vi "Zernike_Mode_Boolean_Selector_v01.vi"(0 "1st  Spherical Aberration":bool, 1 "2nd Spherical Aberration":bool, 2 "Oblique Astigmatism":bool, 3 "Vertical Astigmatism":bool, 4 "Horizontal Coma":bool, 5 "Vertical Coma":bool) -> (14 "ZM 1":i32[](array[numeric]), 15 "ZM 2":i32[](array[numeric]))   [LabVIEW 2015]
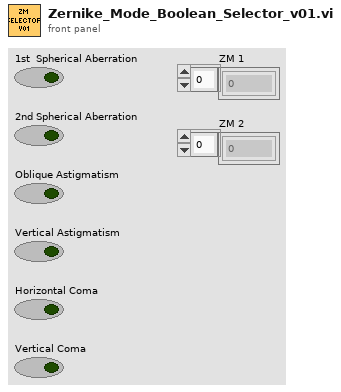
[diagram p1: front panel]
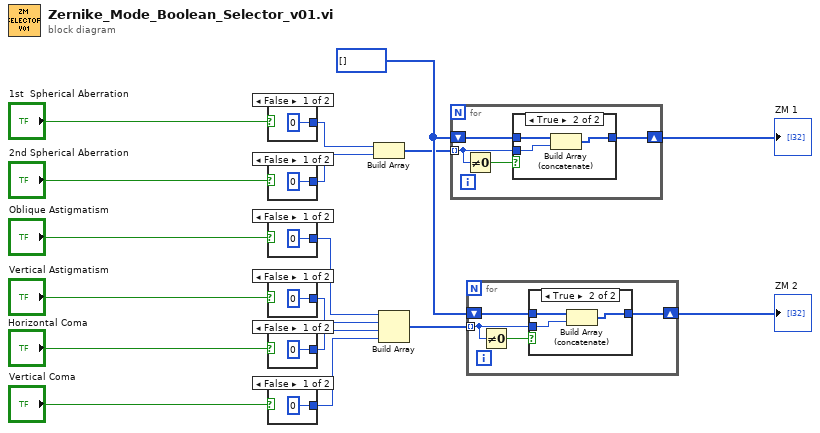
[diagram p0: block diagram]
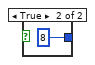
[diagram p4: hidden frame]
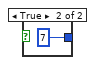
[diagram p5: hidden frame]
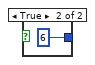
[diagram p6: hidden frame]
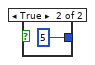
[diagram p7: hidden frame]
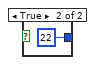
[diagram p8: hidden frame]
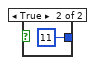
[diagram p9: hidden frame]
diagram:
  w16 = i32[] []
  n1 = case shown="False" "1st  Spherical Aberration" {
    tunnel: [0 11] -> w7
    frame False {
    }
    frame True {
    }
  }
  n2 = case shown="False" "2nd Spherical Aberration" {
    tunnel: [0 22] -> w8
    frame False {
    }
    frame True {
    }
  }
  n3 = case shown="False" "Oblique Astigmatism" {
    tunnel: [0 5] -> w9
    frame False {
    }
    frame True {
    }
  }
  n4 = case shown="False" "Vertical Astigmatism" {
    tunnel: [0 6] -> w10
    frame False {
    }
    frame True {
    }
  }
  n5 = case shown="False" "Horizontal Coma" {
    tunnel: [0 7] -> w11
    frame False {
    }
    frame True {
    }
  }
  n6 = case shown="False" "Vertical Coma" {
    tunnel: [0 8] -> w12
    frame False {
    }
    frame True {
    }
  }
  n7 = Build Array(w7, w8) -> (w13:i32[])
  n8 = Build Array(w9, w10, w11, w12) -> (w17:i32[])
  n9 = for {
    tunnel: w13 -> [w32] mode=indexing
    shift-right: [w30] -> w14
    shift-left: w16 -> [w31]
    n10 = Not Equal To 0?(x=w32) -> (x != 0?=w33:bool)
    n11 = case shown="True" w33 {
      tunnel: w32 -> [_ w37]
      tunnel: w31 -> [w34 w36]
      tunnel: [w34 w35] -> w30
      frame False {
      }
      frame True {
        n12 = Build Array (concatenate)(w36, w37) -> (w35:i32[])
      }
    }
  }
  "ZM 1" <- w14
  n13 = for {
    tunnel: w17 -> [w40] mode=indexing
    shift-right: [w38] -> w15
    shift-left: w16 -> [w39]
    n14 = Not Equal To 0?(x=w40) -> (x != 0?=w41:bool)
    n15 = case shown="True" w41 {
      tunnel: w40 -> [_ w45]
      tunnel: w39 -> [w42 w44]
      tunnel: [w42 w43] -> w38
      frame False {
      }
      frame True {
        n16 = Build Array (concatenate)(w44, w45) -> (w43:i32[])
      }
    }
  }
  "ZM 2" <- w15
